vi "PlinkSSH.vi"() -> ()   [LabVIEW 2012]
panel:
  out "error out":errorcluster
  in  "error in (no error)":errorcluster
  out "standard error":string
  out "standard output":string
  in  "Use Script?":bool
  in  "password":string
  in  "Username":string
  in  "Command(s) to Execute":string="pwd"
  in  "Host":string="130.64.87.197"
  out "command line input":string
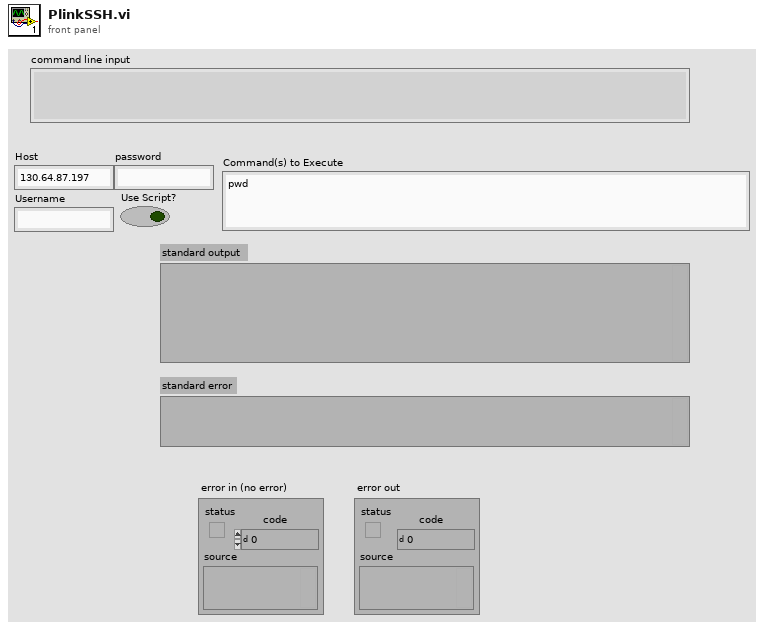
[diagram p1: front panel]
types:
  T1 = enum16{"open", "replace", "create", "open or create", "replace or create", "replace or create with confirmation"}
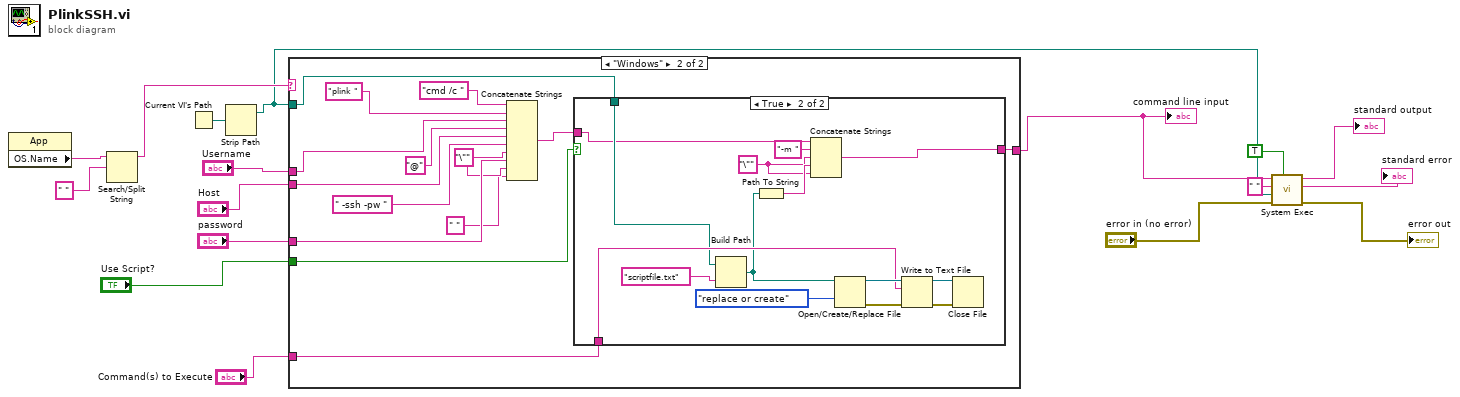
[diagram p0: block diagram]
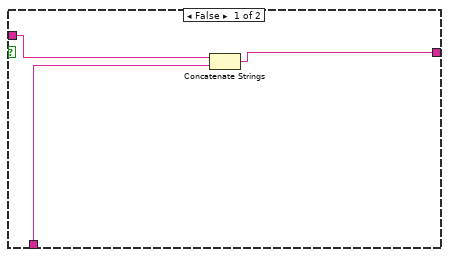
[diagram p3: hidden frame]
diagram:
  n1 = property class="App"() -> ("OS.Name"=w14:string)  [unwired: 2 in, 2 out]
  n2 = Search/Split String(string=w14, search string/char (-)=" ") -> (substring before match=w13:string)  [unwired: 1 in, 2 out]
  n3 = Current VI's Path() -> (path=w17:path)
  n4 = Strip Path(path=w17) -> (stripped path=w4:path)  [unwired: 1 out]
  n5 = case shown="\"Windows\"" w13 {
    tunnel: w4 -> [_ w24]
    tunnel: "Username" -> [_ w30]
    tunnel: "Host" -> [_ w28]
    tunnel: "password" -> [_ w21]
    tunnel: "Use Script?" -> [_ w26]
    tunnel: "Command(s) to Execute" -> [_ w25]
    tunnel: [_ w22] -> w8
    frame "False", Default {
    }
    frame "Windows" {
      w20 = "\"" ("string")
      n6 = Concatenate Strings("cmd /c " ("string"), "plink " ("name or relative path"), w30, "@" ("string"), w28, " -ssh -pw " ("string"), w20, w21, w20, " " ("string")) -> (w23:string)
      n7 = case shown="True" w26 {
        tunnel: w25 -> [w33 w43]
        tunnel: w24 -> [_ w41]
        tunnel: w23 -> [w34 w40]
        tunnel: [w32 w37] -> w22
        frame False {
          n8 = Concatenate Strings(w34, w33) -> (w32:string)
        }
        frame True {
          w35 = "\"" ("string")
          n9 = Build Path(base path=w41, name or relative path="scriptfile.txt" ("Script File Name")) -> (appended path=w38:path)
          n10 = Path To String(path=w38) -> (string=w36:string)
          n11 = Concatenate Strings(w40, "-m " ("string"), w35, w36, w35) -> (w37:string)
          n12 = Open/Create/Replace File(file path (use dialog)=w38, operation (0:open)=T1."replace or create") -> (refnum out=w46:refnum<file>, error out=w45:errorcluster)  [unwired: 4 in, 1 out]
          n13 = Write to Text File(file (use dialog)=w46, text=w43, error in=w45) -> (refnum out=w48:refnum<file>, error out=w47:errorcluster)  [unwired: 2 out]
          n14 = Close File(refnum=w48, error in=w47) -> ()  [unwired: 2 out]
        }
      }
    }
  }
  "command line input" <- w8
  n15 = call <vilib>:"System Exec.vi"("wait until completion? (T)"=TRUE, "error in (no error)"="error in (no error)", "working directory"=w4, "standard input"=" ", "command line"=w8) -> ("error out"=→"error out":errorcluster, "standard error"=→"standard error":string, "standard output"=→"standard output":string)  [unwired: 3 in, 1 out]
